vi "changeToVolt.vi"(8 "error in (no error)":errorcluster, 11 "Electrometer in":refnum<class "Electrometer.lvclass">) -> (0 "error out":errorcluster, 3 "Electrometer out":refnum<class "Electrometer.lvclass">)   [LabVIEW 2016, in "Electrometer.lvclass"]
uses:
  Electrometer.lvclass
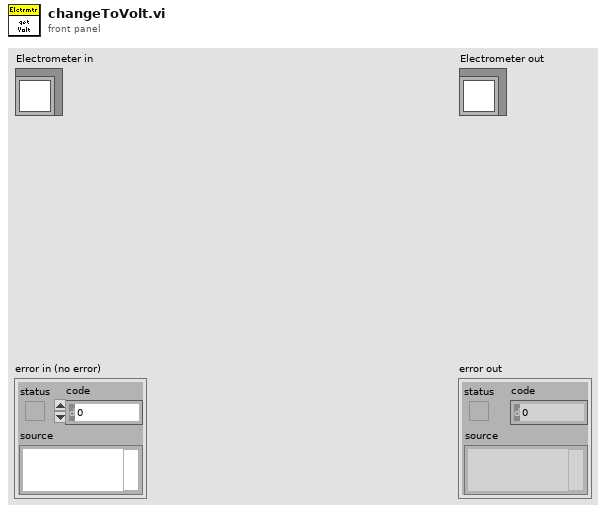
[diagram p1: front panel]
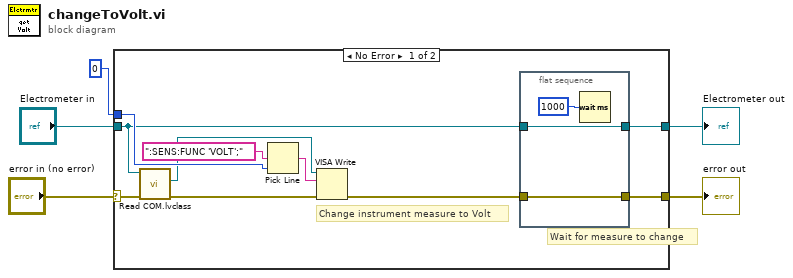
[diagram p0: block diagram]
diagram:
  n1 = case shown="No Error" "error in (no error)" {
    selector: "error in (no error)" -> [w11 w20]
    tunnel: [w6 w20] -> w4
    tunnel: [w8 w19] -> w2
    tunnel: "Electrometer in" -> [w9 w19]
    tunnel: 0 ("Reading Option (0: Latest)") -> [w13 _]
    frame No Error {
      # "Wait for measure to change"
      # "Change instrument measure to Volt"
      n2 = call "Read COM.lvclass.vi"("error in (no error)"=w11, "Electrometer in"=w9) -> ("error out"=w12:errorcluster, "VISA"=w10:refnum<visa-resource-name>)  [unwired: 7 in, 1 out]
      n3 = Pick Line(multi-line string=":SENS:FUNC 'VOLT';", line index=w13) -> (output string=w15:string)  [unwired: 1 in]
      n4 = VISA Write(VISA resource name=w10, write buffer=w15, error in (no error)=w12) -> (error out=w7:errorcluster)  [unwired: 2 out]
      n5 = flat-sequence {
        tunnel: w9 -> [w18]
        tunnel: [w18] -> w8
        tunnel: w7 -> [w17]
        tunnel: [w17] -> w6
        frame #0 {
          n6 = Wait (ms)(milliseconds to wait=u32 1000) -> ()  [unwired: 1 out]
        }
      }
    }
    frame Error {
    }
  }
  "error out" <- w4
  "Electrometer out" <- w2
